vi "Omni-Bus Inject Multi CEXT.vi"(6 "Enable":bool[](array[boolean]), 8 "error in (no error)":errorcluster, 9 "Injected Values":cxt[](array[numeric]), 10 "Tag":string[](array[string]), 11 "Omni_Bus in":refnum<class "Omni_Bus.lvclass">) -> (0 "error out":errorcluster, 3 "Omni_Bus out":refnum<class "Omni_Bus.lvclass">)   [LabVIEW 2021, in "Fault-Injection Bus.lvclass"]
uses:
  Fault-Injection Bus.lvclass
  Omni-Bus/Omni_Bus.lvclass
  Value Type/CEXT/Fault-Injection_CEXT.lvclass
  C:/Program Files (x86)/National Instruments/LabVIEW 2021/vi.lib/TSA/Abstract Data Classes/Abs_Types/Type/Abs_Type.lvclass
  Omni-Bus/Support/FindVar.vi
  <vilib>/TSA/Abstract Data Classes/Abs_Types/Type/Abs_Type.lvclass
  Fault-Injection Bus.lvclass/Fault-Injection Bus.ctl
  C:/Program Files (x86)/National Instruments/LabVIEW 2021/vi.lib/TSA/Abstract Data Classes/Abs_Types/Complex Extended Float/Abs_Complex Extended Float.lvclass
  C:/Program Files (x86)/National Instruments/LabVIEW 2021/vi.lib/TSA/Abstract Data Classes/Abs_Types/Floating Point/Abs_Floating Point.lvclass
  C:/Program Files (x86)/National Instruments/LabVIEW 2021/vi.lib/TSA/Abstract Data Classes/Abs_Types/Numeric/Abs_Numeric.lvclass
  C:/Program Files (x86)/National Instruments/LabVIEW 2021/vi.lib/TSA/Abstract Data Classes/Abs_Types/Value/Abs_Value.lvclass
  C:/TSA/Omni-Bus/Source/Fault-Injection Bus/Support/Interfaces/CEXT/Fault-Injection_CEXT_Type.lvclass
  C:/TSA/Omni-Bus/Source/Fault-Injection Bus/Support/Interfaces/Type/Fault-Injection_Type.lvclass
  C:/TSA/Omni-Bus/Source/Fault-Injection Bus/Support/Value Type/CEXT/Fault-Injection_CEXT.lvclass
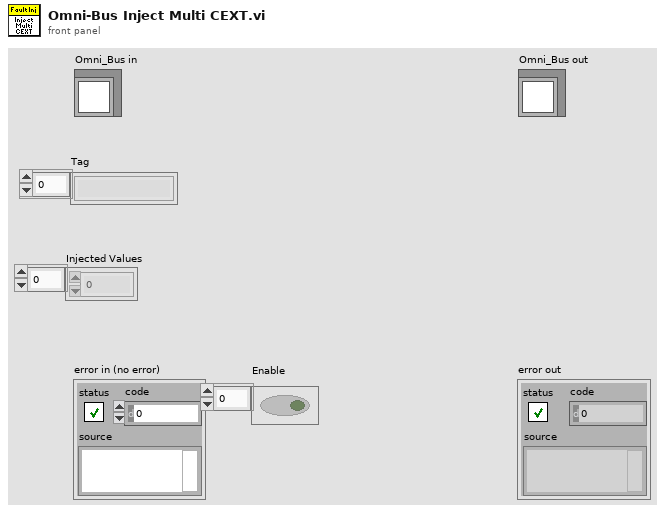
[diagram p1: front panel]
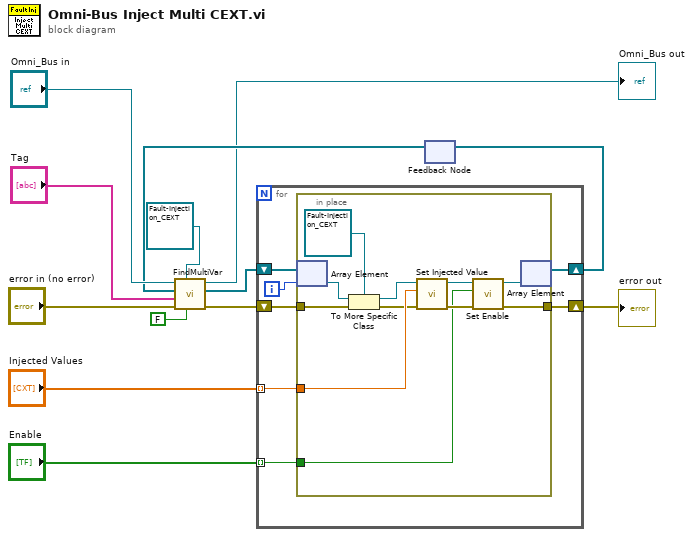
[diagram p0: block diagram]
diagram:
  n1 = feedback #1() -> (w9:refnum<class "Abs_Type.lvclass">[])  [unwired: 1 in]
  n2 = call "FindMultiVar.vi"("Write?"=FALSE, "Abs_Type"=refnum<class "Fault-Injection_CEXT.lvclass"> refnum ("Fault-Injection_Boolean out"), "error in (no error)"="error in (no error)", "Tag"="Tag", "Abs_Type Default"=w9, "Var Bus in"="Omni_Bus in") -> ("error out"=w12:errorcluster, "Abs_Type Found"=w11:refnum<class "Abs_Type.lvclass">[], "Var Bus out"=→"Omni_Bus out":refnum<class "Omni_Bus.lvclass">)  [unwired: 2 in, 1 out]
  n3 = for {
    tunnel: "Injected Values" -> [w20] mode=indexing
    tunnel: "Enable" -> [w19] mode=indexing
    shift-right: [w18] -> w5
    shift-left: w12 -> [w17]
    shift-right: [w15] -> w8
    shift-left: w11 -> [w16]
    i -> [w14]
    n4 = in-place {
      in-place-border: w20 -> [w29]
      in-place-border: w19 -> [w28]
      in-place-border: [w27] -> w18
      in-place-border: w17 -> [w25]
      n5 = in-place-array #2(w16, w14) -> (w22:refnum<class "Abs_Type.lvclass">)
      n6 = To More Specific Class(target class=refnum<class "Fault-Injection_CEXT.lvclass"> refnum ("Fault-Injection_Boolean out"), reference=w22, error in=w25) -> (specific class reference=w23:refnum<class "Fault-Injection_CEXT.lvclass">, error out=w26:errorcluster)
      n7 = call-dynamic "Set Injected Value.vi"("error in (no error)"=w26, "Value"=w29, "Fault-Injection_Boolean in"=w23) -> ("error out"=w31:errorcluster, "Fault-Injection_Boolean out"=w30:refnum<class "Fault-Injection_CEXT.lvclass">)  [unwired: 7 in]
      n8 = call-dynamic "Set Enable.vi"("error in (no error)"=w31, "Enable"=w28, "Fault-Injection_Boolean in"=w30) -> ("error out"=w27:errorcluster, "Fault-Injection_Boolean out"=w21:refnum<class "Fault-Injection_CEXT.lvclass">)  [unwired: 7 in]
      n9 = in-place-array #2(w21) -> (w15:refnum<class "Abs_Type.lvclass">[])  [unwired: 1 out]
    }
  }
  "error out" <- w5
  n10 = feedback-in #1(w8) -> ()
